vi "temperature converter.vi"(8 "Boolean":bool, 11 "Celcius":dbl) -> (3 "Numeric":dbl)   [LabVIEW 2025]
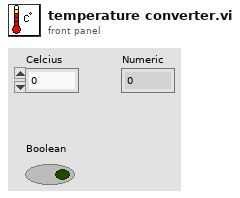
[diagram p1: front panel]
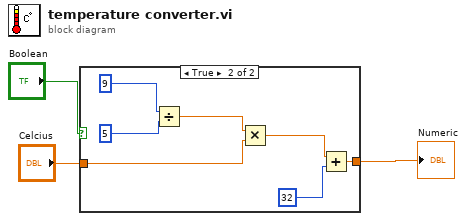
[diagram p0: block diagram]
diagram:
  n1 = case shown="True" "Boolean" {
    tunnel: [w4 w10] -> w1
    tunnel: "Celcius" -> [w4 w8]
    frame False {
    }
    frame True {
      n2 = Divide(x=9, y=5) -> (x/y=w7:dbl)
      n3 = Multiply(x=w7, y=w8) -> (x*y=w11:dbl)
      n4 = Add(x=w11, y=32) -> (x+y=w10:dbl)
    }
  }
  "Numeric" <- w1
